vi "Signed Array Index.vi"(9 "Array Size":i32, 10 "Array Index in":i32) -> (2 "Array Index out":i32)   [LabVIEW 2021, in "Arrays.lvlib"]
doc: "use i[n] (i modulo n) as the resulting index, where i is the input index and n is the number of array element, making it a circular array.\n\nFot instance, to select the last array element, use -1.\n\nUsing i = n results in the firs element to be selected (i -> 0), etc."
uses:
  Arrays.lvlib
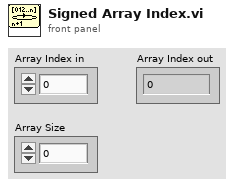
[diagram p1: front panel]
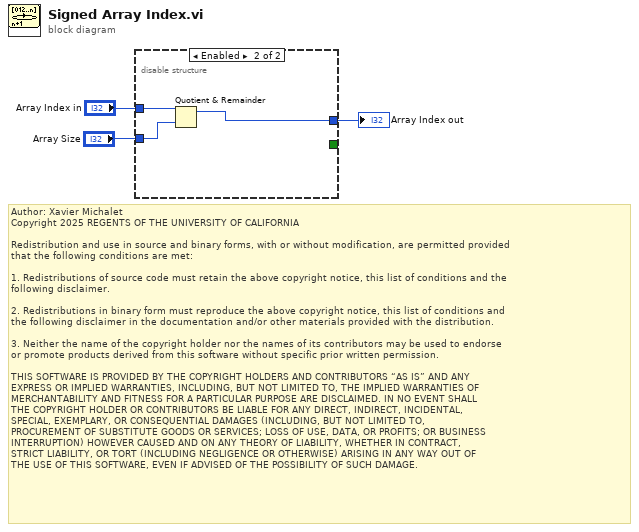
[diagram p0: block diagram]
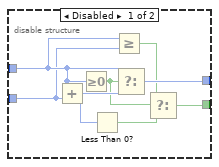
[diagram p2: hidden frame]
diagram:
  # "Author: Xavier Michalet\nCopyright 2025 REGENTS OF THE UNIVERSITY OF CALIFORNIA\n\nRedistribution and use in source and binary forms, with or without modification, are permitted provided\nthat the following conditions are met:\n\n1. Redistributions of source code must retain the above copyright notice, this list of conditions and the\nfollowing disclaimer.\n\n2. Redistributions in binary form must reproduce the above copyright notice, this list of conditions and\nthe following disclaimer in the documentation and/or other materials provided with the distribution.\n\n3. Neither the name of the copyright holder nor the names of its contributors may be used to endorse \nor promote products derived from this software without specific prior written permission.\n\nTHIS SOFTWARE IS PROVIDED BY THE COPYRIGHT HOLDERS AND CONTRIBUTORS “AS IS” AND ANY \nEXPRESS OR IMPLIED WARRANTIES, INCLUDING, BUT NOT LIMITED TO, THE IMPLIED WARRANTIES OF\nMERCHANTABILITY AND FITNESS FOR A PARTICULAR PURPOSE ARE DISCLAIMED. IN NO EVENT SHALL\nTHE COPYRIGHT HOLDER OR CONTRIBUTORS BE LIABLE FOR ANY DIRECT, INDIRECT, INCIDENTAL, \nSPECIAL, EXEMPLARY, OR CONSEQUENTIAL DAMAGES (INCLUDING, BUT NOT LIMITED TO, \nPROCUREMENT OF SUBSTITUTE GOODS OR SERVICES; LOSS OF USE, DATA, OR PROFITS; OR BUSINESS\nINTERRUPTION) HOWEVER CAUSED AND ON ANY THEORY OF LIABILITY, WHETHER IN CONTRACT, \nSTRICT LIABILITY, OR TORT (INCLUDING NEGLIGENCE OR OTHERWISE) ARISING IN ANY WAY OUT OF\nTHE USE OF THIS SOFTWARE, EVEN IF ADVISED OF THE POSSIBILITY OF SUCH DAMAGE."
  n1 = disable-structure shown="Enabled" {
    disable-tunnel: [w11 w12] -> w3
    disable-tunnel: "Array Index in" -> [w10 w14]
    disable-tunnel: "Array Size" -> [w9 w13]
    disable-tunnel: [w4 _] -> _
    frame Disabled {
      n2 = Add(x=w10, y=w9) -> (x+y=w8:i32)
      n3 = Greater Or Equal To 0?(x=w10) -> (x >= 0?=w7:bool)
      n4 = Less Than 0?(x=w8) -> (x < 0?=w5:bool)
      n5 = Greater Or Equal?(x=w10, y=w9) -> (x >= y?=w6:bool)
      n6 = Select(t=w10, s=w7, f=w8) -> (s? t:f=w11:i32)
      n7 = Select(t=w6, s=w7, f=w5) -> (s? t:f=w4:bool)
    }
    frame Enabled {
      n8 = Quotient & Remainder(x=w14, y=w13) -> (x-y*floor(x/y)=w12:i32)  [unwired: 1 out]
    }
  }
  "Array Index out" <- w3
